vi "Update angle chart -- subVI.vi"(8 "error in (no error)":errorcluster, 9 "Val read":dbl, 10 "FCR Mod ID":i32, 11 "Angle chart in":cluster{"Angle":dbl, "Data":dbl}[](array[cluster])) -> (0 "error out":errorcluster, 2 "Position":dbl, 3 "Angle chart out":cluster{"Angle":dbl, "Data":dbl}[](array[cluster]))   [LabVIEW 2020]
uses:
  Newport_FCR100/Libraries/FCR100/FCR100.lvlib
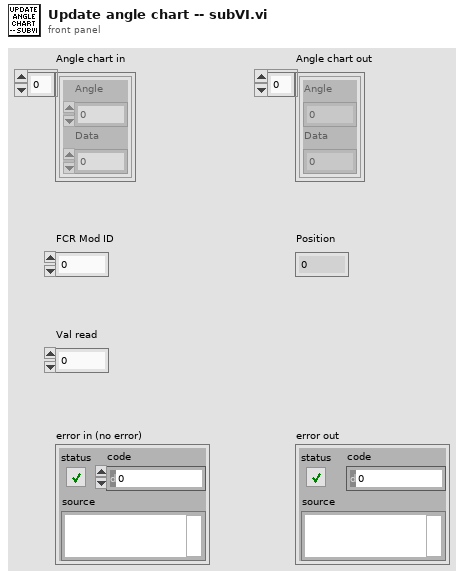
[diagram p1: front panel]
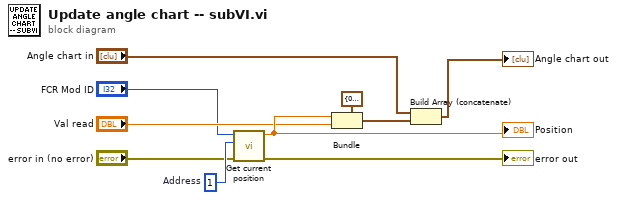
[diagram p0: block diagram]
diagram:
  w8 = u8 1  # Address
  n1 = call "Get current position.vi"("error in"="error in (no error)", "Address"=w8, "Module ID"="FCR Mod ID") -> ("error out"=→"error out":errorcluster, "Position"=w10:dbl)  [unwired: 6 in, 1 out]
  "Position" <- w10
  n2 = Bundle(cluster=cluster{"Angle":dbl, "Data":dbl} {"Angle"=0.0, "Data"=0.0} ("Angle vs V"), "Angle"=w10, "Data"="Val read") -> (w3:cluster{"Angle":dbl, "Data":dbl})
  n3 = Build Array (concatenate)("Angle chart in", w3) -> (→"Angle chart out":cluster{"Angle":dbl, "Data":dbl}[])
